vi "Resize.vi"(10 "Capacity 2^n":u32, 11 "POTTypedCircularBuffer in":refnum<class "ErrorLogBuffer.lvclass">) -> (3 "POTTypedCircularBuffer out":refnum<class "ErrorLogBuffer.lvclass">)   [LabVIEW 2024, in "ErrorLogBuffer.lvclass"]
uses:
  ErrorLogBuffer.lvclass
  ErrorLogBuffer.lvclass/ErrorLogBuffer.ctl
  Type.ctl
  RQMHCore/ErrorReporting/Record/LogRecord.lvclass
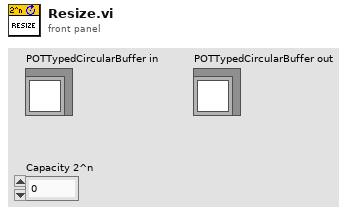
[diagram p1: front panel]
types:
  T1 = typedef "ErrorLogBuffer.lvclass/Type.ctl" = refnum<class "LogRecord.lvclass">
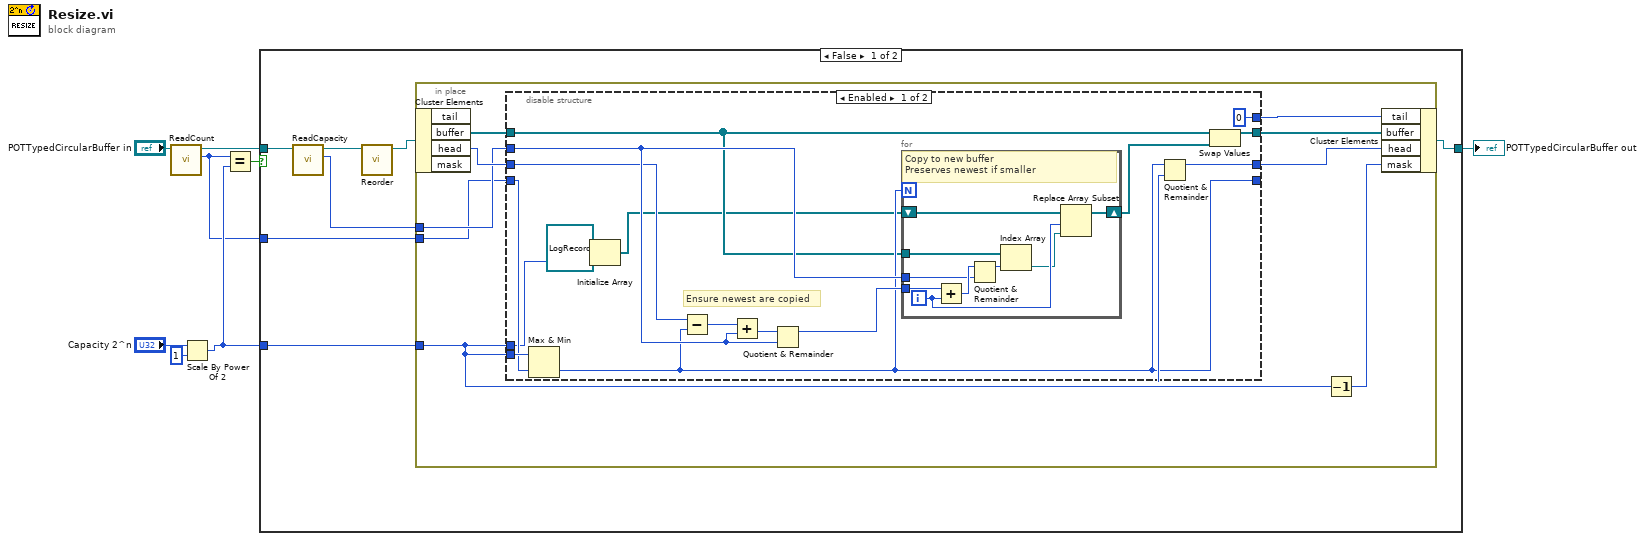
[diagram p0: block diagram]
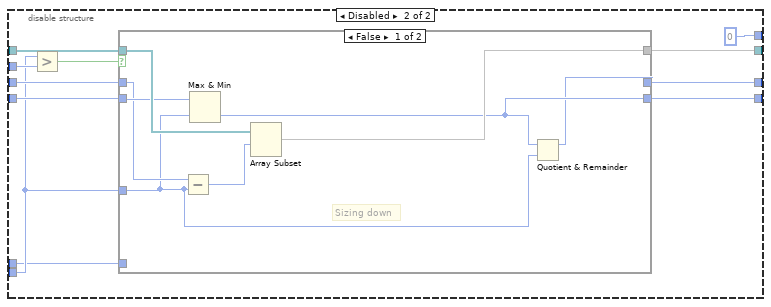
[diagram p2: hidden frame]
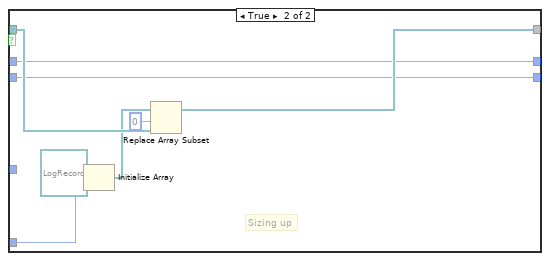
[diagram p3: hidden frame]
diagram:
  n1 = call "ReadCount.vi"("POTTypedCircularBuffer in"="POTTypedCircularBuffer in") -> ("count"=w1:i32, "POTTypedCircularBuffer out"=w5:refnum<class "ErrorLogBuffer.lvclass">)  [unwired: 9 in]
  n2 = Scale By Power Of 2(n="Capacity 2^n", x=1) -> (x*2^n=w2:i32)
  n3 = Equal?(x=w1, y=w2) -> (x = y?=w7:bool)
  n4 = case shown="False" w7 {
    tunnel: [w14 w77] -> w6
    tunnel: w5 -> [w10 w77]
    tunnel: w2 -> [w15 _]
    tunnel: w1 -> [w12 _]
    frame False {
      n5 = call "ReadCapacity.vi"("POTTypedCircularBuffer in"=w10) -> ("capacity"=w9:i32, "POTTypedCircularBuffer out"=w11:refnum<class "ErrorLogBuffer.lvclass">)  [unwired: 9 in]
      n6 = call "Reorder.vi"("POTTypedCircularBuffer in"=w11) -> ("POTTypedCircularBuffer out"=w13:refnum<class "ErrorLogBuffer.lvclass">)  [unwired: 10 in]
      n7 = in-place {
        in-place-border: w15 -> [w19]
        in-place-border: w12 -> [w16]
        in-place-border: w9 -> [w17]
        n8 = in-place-cluster #1(w13) -> ("buffer"=w21:T1[], "head"=w20:i32)  [unwired: 2 out]
        n9 = disable-structure shown="Enabled" {
          disable-tunnel: [w40 w56] -> w24
          disable-tunnel: w17 -> [w37 w59]
          disable-tunnel: [w35 w54] -> w23
          disable-tunnel: w19 -> [w34 w51]
          disable-tunnel: [0 ("tail") 0 ("tail")] -> w22
          disable-tunnel: [w32 w52] -> _
          disable-tunnel: w16 -> [w31 w53]
          disable-tunnel: w21 -> [w30 w57]
          disable-tunnel: w20 -> [w29 w55]
          disable-tunnel: w19 -> [w26 w50]
          frame Enabled {
            # "Ensure newest are copied"
            n10 = Max & Min(x=w34, y=w31) -> (min(x,y)=w32:i32)  [unwired: 1 out]
            n11 = Initialize Array(T1 refnum ("Type"), w26) -> (w25:T1[])
            n12 = Subtract(x=w29, y=w32) -> (x-y=w39:i32)
            n13 = Add(x=w39, y=w37) -> (x+y=w38:i32)
            n14 = Quotient & Remainder(x=w38, y=w37) -> (x-y*floor(x/y)=w36:i32)  [unwired: 1 out]
            n15 = for {
              N: w32 -> [_]
              tunnel: w30 -> [w49]
              tunnel: w36 -> [w48]
              tunnel: w37 -> [w46]
              shift-right: [w44] -> w28
              shift-left: w25 -> [w45]
              i -> [w42]
              # "Copy to new buffer\nPreserves newest if smaller"
              n16 = Add(x=w48, y=w42) -> (x+y=w47:i32)
              n17 = Quotient & Remainder(x=w47, y=w46) -> (x-y*floor(x/y)=w43:i32)  [unwired: 1 out]
              n18 = Index Array(array=w49, index=w43) -> (element=w41:T1)
              n19 = Replace Array Subset(array=w45, new element=w41, index=w42) -> (w44:T1[])
            }
            n20 = Quotient & Remainder(x=w32, y=w34) -> (x-y*floor(x/y)=w35:i32)  [unwired: 1 out]
            n21 = Swap Values(12:w30, 14:w28) -> (1:w40:T1[])  [unwired: 1 in, 1 out]
          }
          frame Disabled {
            n22 = Greater?(x=w51, y=w59) -> (0:w58:bool)
            n23 = case shown="False" w58 {
              tunnel: w57 -> [w68 w76]
              tunnel: [w67 w75] -> w56
              tunnel: w55 -> [w65 w74]
              tunnel: [w61 w74] -> w54
              tunnel: w53 -> [w66 w73]
              tunnel: [w63 w73] -> w52
              tunnel: w51 -> [w64 _]
              tunnel: w50 -> [_ w70]
              frame False {
                # "Sizing down"
                n24 = Subtract(x=w65, y=w64) -> (x-y=w62:i32)
                n25 = Max & Min(x=w66, y=w64) -> (min(x,y)=w63:i32)  [unwired: 1 out]
                n26 = Array Subset(array=w68, index=w62) -> (w67:T1[])  [unwired: 1 in]
                n27 = Quotient & Remainder(x=w63, y=w64) -> (x-y*floor(x/y)=w61:i32)  [unwired: 1 out]
              }
              frame True {
                # "Sizing up"
                n28 = Initialize Array(T1 refnum ("Type"), w70) -> (w69:T1[])
                n29 = Replace Array Subset(array=w69, new element=w76, index=0) -> (w75:T1[])
              }
            }
          }
        }
        n30 = Decrement(x=w19) -> (x-1=w18:i32)
        n31 = in-place-cluster #1("tail"=w22, "buffer"=w24, "head"=w23, "mask"=w18) -> (w14:refnum<class "ErrorLogBuffer.lvclass">)
      }
    }
    frame True {
    }
  }
  "POTTypedCircularBuffer out" <- w6
